vi "trio_wait_idle.vi"(7 "Timeout":u32=10000, 8 "error in":errorcluster, 9 "Poll delay":u32=50, 10 "Axis enable":bool[](array[boolean]), 11 "Trio ref in":refnum<k7>) -> (0 "error out":errorcluster, 2 "Moving axes":bool[](array[boolean]), 3 "Trio ref out":refnum<k7>)   [LabVIEW 2017]
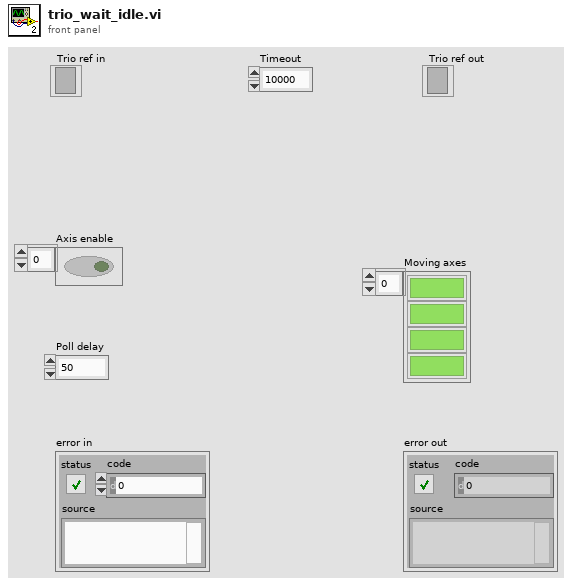
[diagram p1: front panel]
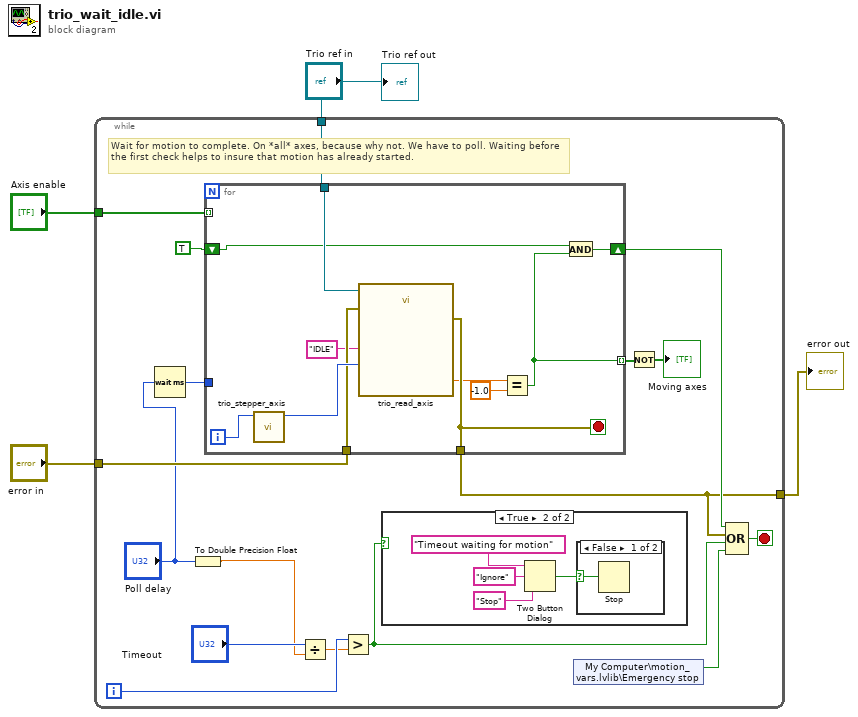
[diagram p0: block diagram]
diagram:
  n1 = while {
    tunnel: "Axis enable" -> [w21]
    tunnel: "error in" -> [w20]
    tunnel: "Trio ref in" -> [w19]
    tunnel: [w15] -> w4
    i -> [w11]
    stop <- w17 stop-if-true
    # "Wait for motion to complete. On *all* axes, because why not. We have to poll. Waiting before the first check helps to insure that motion has already started."
    n2 = Wait (ms)(milliseconds to wait="Poll delay") -> (millisecond timer value=w14:u32)
    n3 = To Double Precision Float(number="Poll delay") -> (double precision float=w5:dbl)
    n4 = for {
      tunnel: w21 -> [_] mode=indexing
      tunnel: w20 -> [w35]
      tunnel: w19 -> [w34]
      tunnel: [w32] -> w15
      shift-right: [w29] -> w16
      shift-left: TRUE -> [w28]
      tunnel: w14 -> [_]
      tunnel: [w27] -> w7 mode=indexing
      i -> [w37]
      stop <- w32 stop-if-true
      n5 = call "trio_stepper_axis.vi"("Encoder axis"=w37) -> ("Stepper axis"=w36:i32)  [unwired: 10 in]
      n6 = call "trio_read_axis.vi"("Axis"=w36, "error in (no error)"=w35, "Variable"="IDLE", "reference in"=w34) -> ("error out"=w32:errorcluster, "Value"=w31:dbl)  [unwired: 5 in, 1 out]
      n7 = Equal?(x=w31, y=-1.0) -> (x = y?=w27:bool)
      n8 = And(x=w28, y=w27) -> (x .and. y?=w29:bool)
    }
    n9 = Divide(x="Timeout", y=w5) -> (x/y=w10:dbl)
    n10 = Greater?(x=w11, y=w10) -> (0:w8:bool)
    n11 = case shown="True" w8 {
      frame False {
      }
      frame True {
        n12 = Two Button Dialog(message="Timeout waiting for motion", 1:"Stop" ("F button name (\"Cancel\")"), 2:"Ignore" ("T button name (\"OK\")")) -> (T button?=w22:bool)
        n13 = case shown="False" w22 {
          selector: w22 -> [w26 _]
          frame False {
            n14 = Stop(stop? (T)=w26) -> ()
          }
          frame True {
          }
        }
      }
    }
    n15 = shared-variable "My Computer\\motion_vars.lvlib\\Emergency stop"() -> (w9:bool)  [unwired: 1 in, 1 out]
    n16 = Not(x=w7) -> (.not. x?=→"Moving axes":bool[])
    n17 = Compound Arithmetic op=OR(w16, w15, w8, w9) -> (w17:bool)
  }
  "error out" <- w4
  "Trio ref out" <- "Trio ref in"
